vi "SUB_TelnetLogIN.vi"() -> (0 "Pass ?":bool, 1 "telnet connection":T1)   [LabVIEW 2011]
doc: "The Telnet Line Client VI uses the Telnet VIs to simulate a simple Telnet Window."
uses:
  <vilib>/addons/internet/telnet/telnet.llb/Telnet Session.ctl
  Instance           5 23Saved   SUB_TelnetLogIN .vi
  Instance           9 23Saved   SUB_TelnetLogIN .vi
  Instance          10 23Saved   SUB_TelnetLogIN .vi
  <vilib>/addons/internet/NI_InternetTK_Core_VIs.lvlib
panel:
  out "Setting OK?":bool
  out "TelnetPassword":string
  out "Telnet ID":string
  out "mobileIP":string
  out "text":string
  out "data out":string
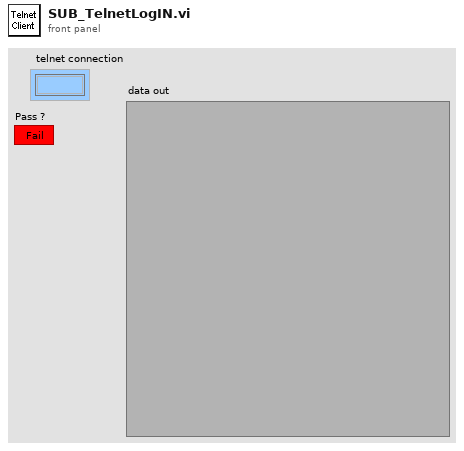
[diagram p1: front panel]
types:
  T1 = typedef "Telnet Session.ctl" = refnum<k1>
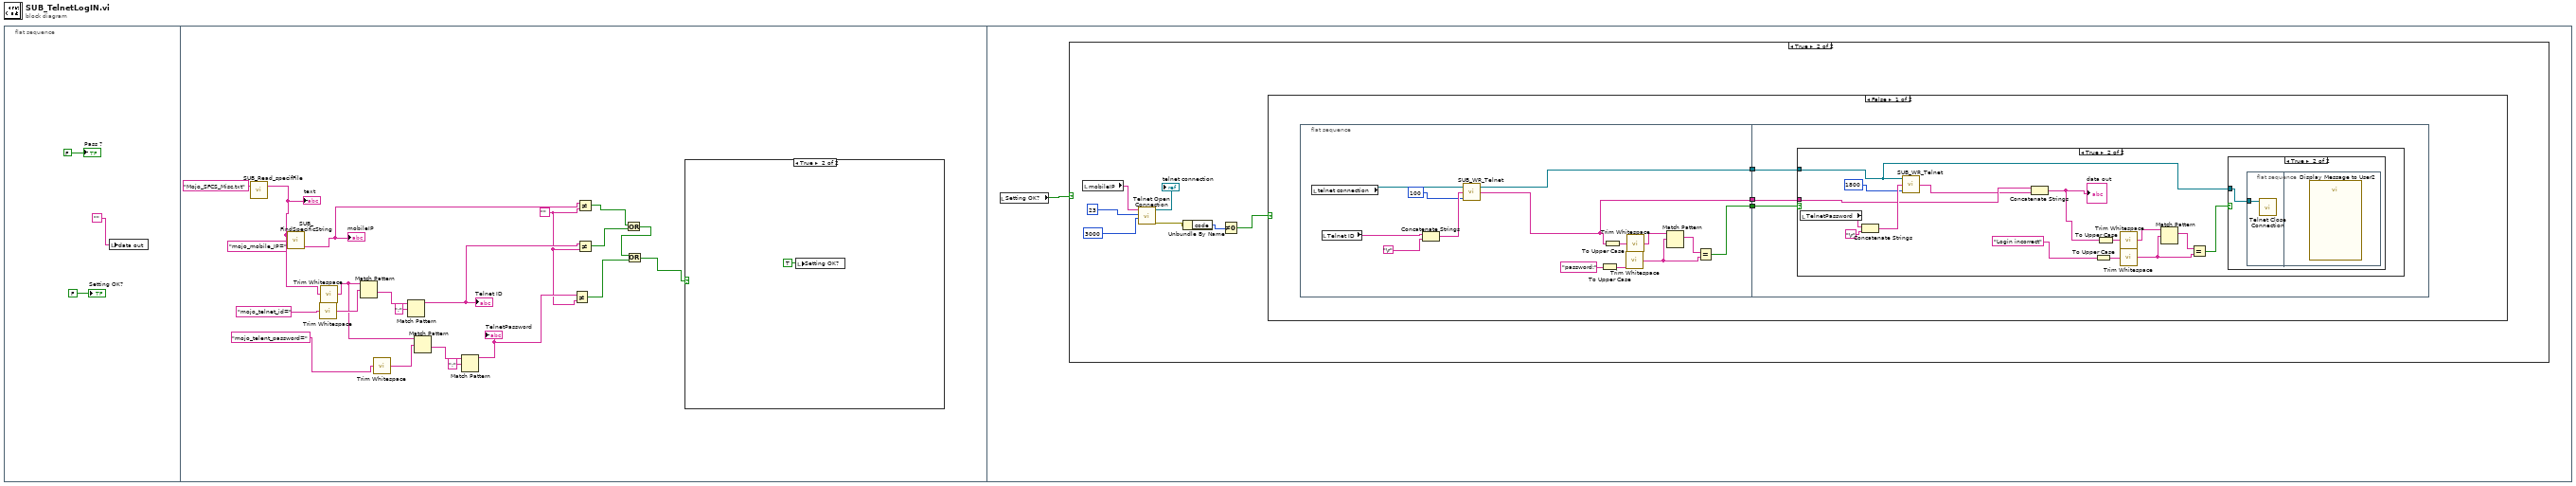
[diagram p0: block diagram]
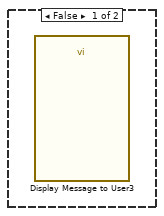
[diagram p2: hidden frame]
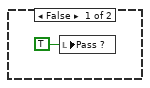
[diagram p5: hidden frame]
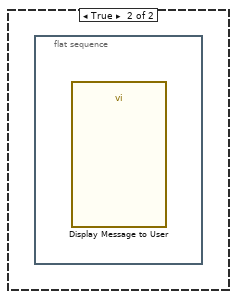
[diagram p6: hidden frame]
diagram:
  n1 = flat-sequence {
    frame #0 {
      n2 = local write "data out"("") -> ()
      "Pass ?" <- FALSE
      "Setting OK?" <- FALSE
    }
    frame #1 {
      w9 = ""
      n3 = call "SUB_Read_specifFile.vi"("name or relative path"="Mojo_SFCS_Misc.txt") -> ("text"=w21:string)  [unwired: 1 in, 1 out]
      "text" <- w21
      n4 = call "SUB_FindSpecificString.vi"("Find this String"="mojo_mobile_IP=", "String data"=w21) -> ("before \"; \" string"=w12:string)  [unwired: 2 in, 1 out]
      "mobileIP" <- w12
      n5 = call <vilib>:"Trim Whitespace.vi"("string"="mojo_telnet_id=") -> ("trimmed string"=w22:string)  [unwired: 1 in]
      n6 = call <vilib>:"Trim Whitespace.vi"("string"=w21) -> ("trimmed string"=w13:string)  [unwired: 1 in]
      n7 = Match Pattern(string=w13, regular expression=w22) -> (after substring=w19:string)  [unwired: 1 in, 3 out]
      n8 = call <vilib>:"Trim Whitespace.vi"("string"="mojo_telent_password=") -> ("trimmed string"=w17:string)  [unwired: 1 in]
      n9 = Match Pattern(string=w19, regular expression=";") -> (before substring=w11:string)  [unwired: 1 in, 3 out]
      "Telnet ID" <- w11
      n10 = Match Pattern(string=w13, regular expression=w17) -> (after substring=w16:string)  [unwired: 1 in, 3 out]
      n11 = Match Pattern(string=w16, regular expression=";") -> (before substring=w10:string)  [unwired: 1 in, 3 out]
      "TelnetPassword" <- w10
      n12 = Not Equal?(x=w10, y=w9) -> (x != y?=w5:bool)
      n13 = Not Equal?(x=w12, y=w9) -> (x != y?=w8:bool)
      n14 = Not Equal?(x=w11, y=w9) -> (x != y?=w7:bool)
      n15 = Or(x=w8, y=w7) -> (x .or. y?=w6:bool)
      n16 = Or(x=w6, y=w5) -> (x .or. y?=w4:bool)
      n17 = case shown="True" w4 {
        frame False {
          n18 = call "Display Message to User3"() -> ()  [unwired: 10 in, 2 out]
        }
        frame True {
          n19 = local write "Setting OK?"(TRUE ("Setting OK?")) -> ()
        }
      }
    }
    frame #2 {
      n20 = local read "Setting OK?"() -> (w26:bool)
      n21 = case shown="True" w26 {
        frame False {
        }
        frame True {
          n22 = local read "mobileIP"() -> (w27:string)
          n23 = call <vilib>:"Telnet Open Connection.vi"("timeout ms (60000)"=3000, "remote port (23)"=u16 23, "address"=w27) -> ("error out"=w30:errorcluster, "telnet connection"=→"telnet connection":T1)  [unwired: 7 in]
          n24 = Unbundle By Name(w30) -> ("code"=w29:i32)
          n25 = Not Equal To 0?(x=w29) -> (x != 0?=w28:bool)
          n26 = case shown="False" w28 {
            frame False {
              n27 = flat-sequence {
                tunnel: [w41] -> w36
                tunnel: [w40] -> w35
                tunnel: [w39] -> w34
                tunnel: w36 -> [w53]
                tunnel: w35 -> [w52]
                tunnel: w34 -> [w51]
                frame #0 {
                  n28 = local read "telnet connection"() -> (w43:T1)
                  n29 = local read "Telnet ID"() -> (w37:string)
                  n30 = Concatenate Strings(w37, "\r") -> (w44:string)
                  n31 = call "SUB_WR_Telnet.vi"("timeout ms"=100, "data in"=w44, "telnet connection"=w43) -> ("data out"=w39:string, "telnet connection out"=w40:T1)  [unwired: 1 in]
                  n32 = To Upper Case(1:"password:" ("string")) -> (0:w49:string)
                  n33 = To Upper Case(1:w39) -> (0:w50:string)
                  n34 = call <vilib>:"Trim Whitespace.vi"("string"=w49) -> ("trimmed string"=w45:string)  [unwired: 1 in]
                  n35 = call <vilib>:"Trim Whitespace.vi"("string"=w50) -> ("trimmed string"=w48:string)  [unwired: 1 in]
                  n36 = Match Pattern(string=w48, regular expression=w45) -> (match substring=w46:string)  [unwired: 1 in, 3 out]
                  n37 = Equal?(x=w46, y=w45) -> (x = y?=w41:bool)
                }
                frame #1 {
                  n38 = case shown="True" w53 {
                    tunnel: w52 -> [_ w54]
                    tunnel: w51 -> [_ w66]
                    frame False {
                    }
                    frame True {
                      n39 = local read "TelnetPassword"() -> (w55:string)
                      n40 = Concatenate Strings(w55, "\r") -> (w68:string)
                      n41 = call "SUB_WR_Telnet.vi"("timeout ms"=1800, "data in"=w68, "telnet connection"=w54) -> ("data out"=w65:string)  [unwired: 1 in, 1 out]
                      n42 = Concatenate Strings(w66, w65) -> (w58:string)
                      "data out" <- w58
                      n43 = To Upper Case(1:"Login incorrect") -> (0:w62:string)
                      n44 = To Upper Case(1:w58) -> (0:w63:string)
                      n45 = call <vilib>:"Trim Whitespace.vi"("string"=w62) -> ("trimmed string"=w59:string)  [unwired: 1 in]
                      n46 = call <vilib>:"Trim Whitespace.vi"("string"=w63) -> ("trimmed string"=w61:string)  [unwired: 1 in]
                      n47 = Match Pattern(string=w61, regular expression=w59) -> (match substring=w60:string)  [unwired: 1 in, 3 out]
                      n48 = Equal?(x=w60, y=w59) -> (x = y?=w56:bool)
                      n49 = case shown="True" w56 {
                        tunnel: w54 -> [_ w70]
                        frame False {
                          n50 = local write "Pass ?"(TRUE ("Pass ?")) -> ()
                        }
                        frame True {
                          n51 = flat-sequence {
                            tunnel: w70 -> [w71]
                            frame #0 {
                              n52 = call <vilib>:"Telnet Close Connection.vi"("telnet connection"=w71) -> ()  [unwired: 9 in, 2 out]
                            }
                            frame #1 {
                              n53 = call "Display Message to User2"() -> ()  [unwired: 10 in, 2 out]
                            }
                          }
                        }
                      }
                    }
                  }
                }
              }
            }
            frame True {
              n54 = flat-sequence {
                frame #0 {
                  n55 = call "Display Message to User"() -> ()  [unwired: 10 in, 2 out]
                }
              }
            }
          }
        }
      }
    }
  }
